vi "Close File.vi"(8 "error in (no error)":errorcluster, 11 "ConfigFile in":refnum<class "ConfigFile.lvclass">) -> (0 "error out":errorcluster)   [LabVIEW 2017, in "ImportExport.lvlib"]
uses:
  ImportExport.lvlib
  ConfigFile/ConfigFile.lvclass
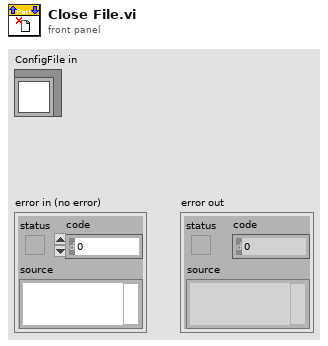
[diagram p1: front panel]
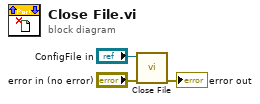
[diagram p0: block diagram]
diagram:
  n1 = call-dynamic "Close File.vi"("error in (no error)"="error in (no error)", "ConfigFile in"="ConfigFile in") -> ("error out"=→"error out":errorcluster)  [unwired: 9 in]
